vi "MultiTimer.vi"(9 "Timer Action (Check)":T1, 11 "Timeout (ms)":u32=60000) -> (1 "Elapsed Time (ms)":u32, 3 "Time Elapsed?":bool)   [LabVIEW 2011]
doc: "Resettable Timer VI\n\n<b>Timeout (ms)</b> The length of time for the timer to mark.\n\n<b>Timer Action (Check)</b> The action to take:\n<b>Check</b>\n<b>Start</b>\n<b>Pause</b>\n<b>Resume</b>\n<b>Stop</b>\n\n<b>Time Elapsed?</b> Indicator of whether the time has elapsed.\n<b>Elapsed Time (ms)</b> Time in milliseconds that have elapsed thus far.\n\n\nVersion 1.0 - 10/21/2009\n\nPhaeron, Inc.\nwww.phaeron.com\ninfo@phaeron.com"
uses:
  TimerAction.ctl
panel:
  in  "Timer#":u8
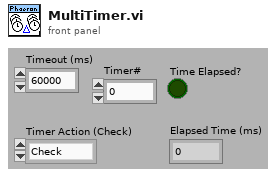
[diagram p1: front panel]
types:
  T1 = typedef "TimerAction.ctl" = enum16{"Check", "Start", "Pause", "Resume", "Stop", "Restart", "Init All"}
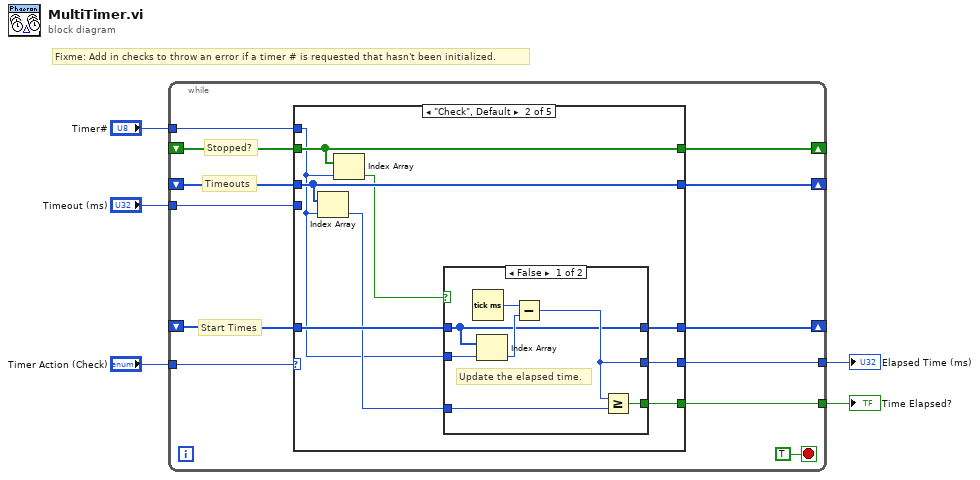
[diagram p0: block diagram]
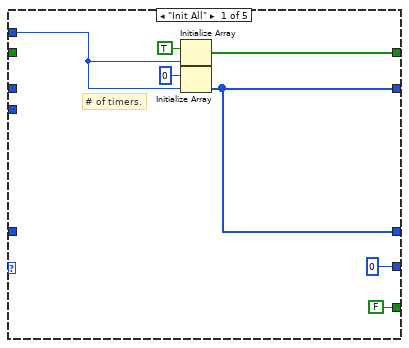
[diagram p2: hidden frame]
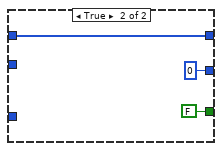
[diagram p3: hidden frame]
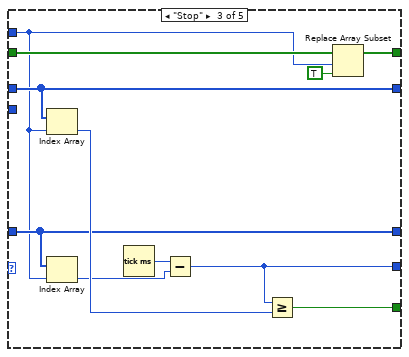
[diagram p4: hidden frame]
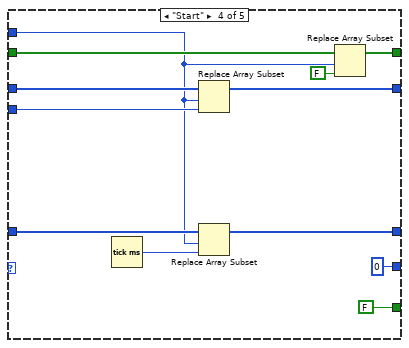
[diagram p5: hidden frame]
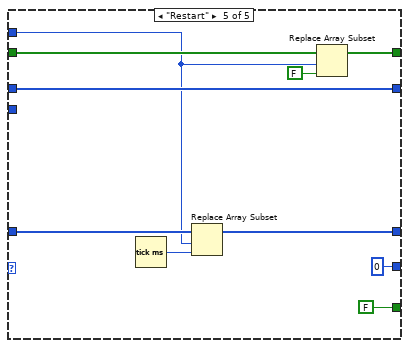
[diagram p6: hidden frame]
diagram:
  # "Fixme: Add in checks to throw an error if a timer # is requested that hasn't been initialized."
  n1 = while {
    tunnel: "Timer Action (Check)" -> [w16]
    tunnel: "Timeout (ms)" -> [w15]
    shift-right: [w14] -> _
    shift-left: _ -> [w13]
    shift-right: [w12] -> _
    shift-left: _ -> [w11]
    tunnel: [w10] -> w3
    tunnel: [w9] -> w2
    shift-right: [w8] -> _
    shift-left: _ -> [w7]
    tunnel: "Timer#" -> [w6]
    stop <- TRUE stop-if-true
    # "Stopped?"
    # "Start Times"
    # "Timeouts"
    n2 = case shown="\"Check\", Default" w16 {
      tunnel: w15 -> [_ _ _ w60 _]
      tunnel: [w23 w30 w52 w59 w74] -> w14
      tunnel: w13 -> [_ w30 w52 w61 w74]
      tunnel: [w23 w26 w50 w64 w72] -> w12
      tunnel: w11 -> [_ w31 w50 w62 w71]
      tunnel: [u32 0 ("element") w33 w44 u32 0 u32 0] -> w10
      tunnel: [FALSE w32 w53 FALSE FALSE] -> w9
      tunnel: [w19 w28 w47 w57 w69] -> w8
      tunnel: w7 -> [_ w28 w48 w58 w70]
      tunnel: w6 -> [w18 w25 w45 w55 w67]
      frame "Init All" {
        # "# of timers."
        n3 = Initialize Array(TRUE, w18) -> (w19:bool[])
        n4 = Initialize Array(u32 0 ("element"), w18) -> (w23:u32[])
      }
      frame "Check", Default {
        n5 = Index Array(array=w30, index=w25) -> (element=w29:u32)
        n6 = Index Array(array=w28, index=w25) -> (element=w27:bool)
        n7 = case shown="False" w27 {
          tunnel: [w40 u32 0] -> w33
          tunnel: [w39 FALSE] -> w32
          tunnel: w31 -> [w35 w41]
          tunnel: w29 -> [w38 _]
          tunnel: [w35 w41] -> w26
          tunnel: w25 -> [w34 _]
          frame False {
            # "Update the elapsed time."
            n8 = Tick Count (ms)() -> (millisecond timer value=w37:u32)
            n9 = Index Array(array=w35, index=w34) -> (element=w36:u32)
            n10 = Subtract(x=w37, y=w36) -> (x-y=w40:u32)
            n11 = Greater Or Equal?(x=w40, y=w38) -> (x >= y?=w39:bool)
          }
          frame True {
          }
        }
      }
      frame "Stop" {
        n12 = Index Array(array=w52, index=w45) -> (element=w51:u32)
        n13 = Index Array(array=w50, index=w45) -> (element=w49:u32)
        n14 = Tick Count (ms)() -> (millisecond timer value=w54:u32)
        n15 = Subtract(x=w54, y=w49) -> (x-y=w44:u32)
        n16 = Greater Or Equal?(x=w44, y=w51) -> (x >= y?=w53:bool)
        n17 = Replace Array Subset(array=w48, new element=TRUE, index=w45) -> (w47:bool[])
      }
      frame "Start" {
        n18 = Tick Count (ms)() -> (millisecond timer value=w63:u32)
        n19 = Replace Array Subset(array=w61, new element=w60, index=w55) -> (w59:u32[])
        n20 = Replace Array Subset(array=w62, new element=w63, index=w55) -> (w64:u32[])
        n21 = Replace Array Subset(array=w58, new element=FALSE, index=w55) -> (w57:bool[])
      }
      frame "Restart" {
        n22 = Tick Count (ms)() -> (millisecond timer value=w73:u32)
        n23 = Replace Array Subset(array=w71, new element=w73, index=w67) -> (w72:u32[])
        n24 = Replace Array Subset(array=w70, new element=FALSE, index=w67) -> (w69:bool[])
      }
    }
  }
  "Elapsed Time (ms)" <- w3
  "Time Elapsed?" <- w2
